vi "AndorLiveMode.vi"(8 "error in (no error)":errorcluster, 11 "Image Name":string="untitled") -> (0 "error out":errorcluster, 3 "Image":T1(plugin-control))   [LabVIEW 2018]
uses:
  <vilib>/vision/NI_Vision_Development_Module.lvlib
  <userlib>/Andor SDK/Andor SDK.lvlib
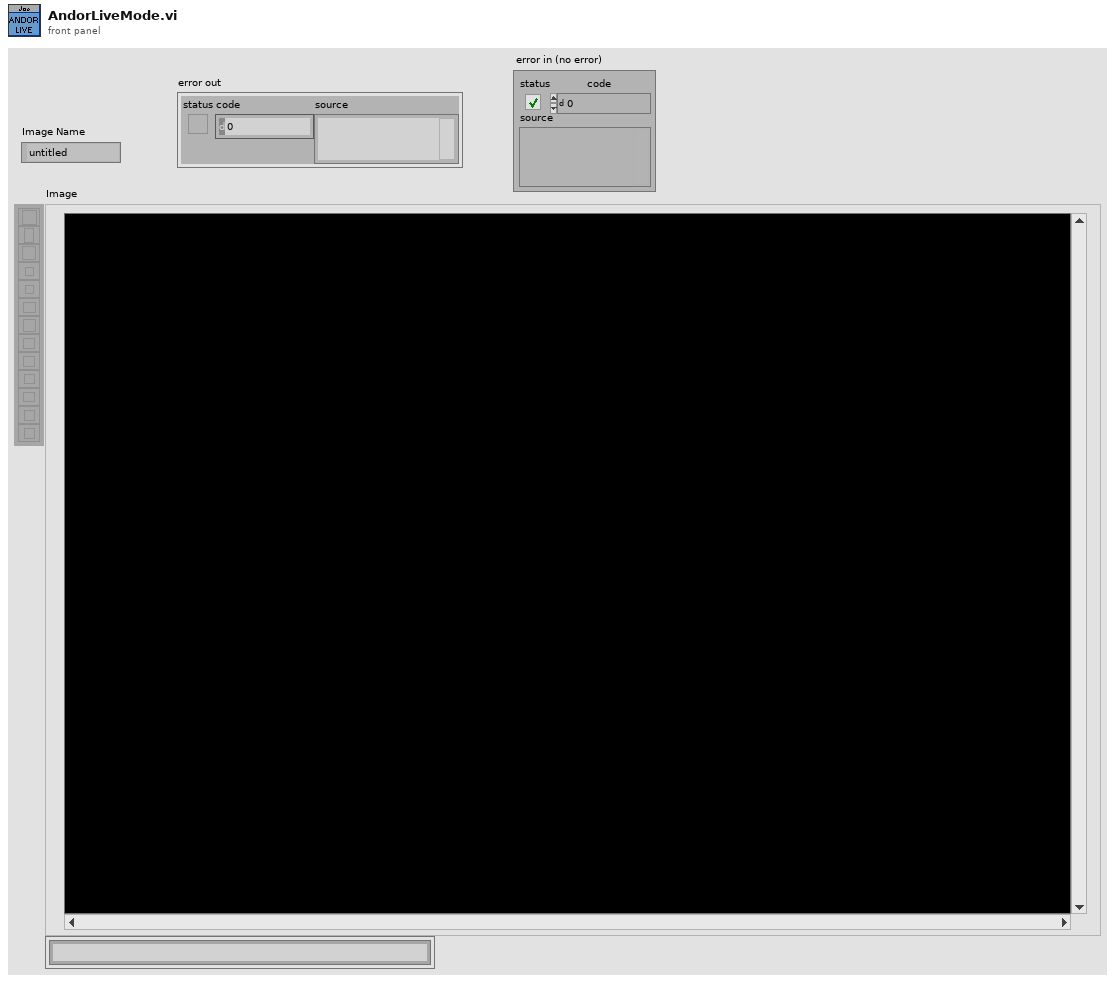
[diagram p1: front panel]
types:
  T1 = typedef "IMAQ Image.ctl" = refnum<image>
  T2 = typedef "Image Type" = u32
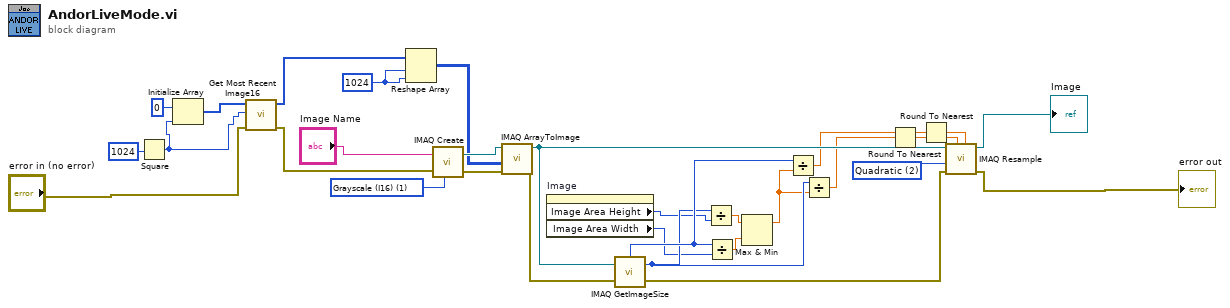
[diagram p0: block diagram]
diagram:
  w13 = u32 2 items=["Zero Order", "Bi-Linear", "Quadratic", "Cubic Spline"] ("Interpolation Type")
  w25 = T2 1 items=["Grayscale (U8)", "Grayscale (I16)", "Grayscale (SGL)", "Complex (CSG)", "RGB (U32)", "HSL (U32)", "RGB (U64)", "Grayscale (U16)"] ("Image Type")
  w26 = 1024 ("dimension size")
  n1 = Square(x=1024) -> (x^2=w11:i32)
  n2 = Initialize Array(0 ("element"), w11) -> (w8:i32[])
  n3 = call <userlib>:"Get Most Recent Image16.vi"("error in (no error)"="error in (no error)", "size"=w11, "arr"=w8) -> ("error out"=w10:errorcluster, "arr out"=w9:u16[])  [unwired: 6 in, 1 out]
  n4 = Reshape Array(w9, w26, w26) -> (w22:u16[][])
  n5 = call "IMAQ Create"("Image Name"="Image Name", "Image Type"=w25, "error in (no error)"=w10) -> ("New Image"=w24:T1, "error out"=w23:errorcluster)  [unwired: 2 in]
  n6 = call "IMAQ ArrayToImage"("error in (no error)"=w23, "Image Pixels (I16)"=w22, "Image"=w24) -> ("error out"=w19:errorcluster, "Image Out"=w15:T1)  [unwired: 7 in]
  n7 = property on="Image" class="ImageControl"() -> ("Image Area Height"=w5:u32, "Image Area Width"=w12:u32)  [unwired: 2 in, 2 out]
  n8 = call "IMAQ GetImageSize"("Image"=w15, "error in (no error)"=w19) -> ("Y Resolution"=w17:i32, "X Resolution"=w18:i32, "error out"=w14:errorcluster)  [unwired: 2 in]
  n9 = Divide(x=w17, y=w5) -> (x/y=w21:dbl)
  n10 = Divide(x=w18, y=w12) -> (x/y=w20:dbl)
  n11 = Max & Min(x=w21, y=w20) -> (max(x,y)=w16:dbl)  [unwired: 1 out]
  n12 = Divide(x=w18, y=w16) -> (x/y=w3:dbl)
  n13 = Divide(x=w17, y=w16) -> (x/y=w4:dbl)
  n14 = Round To Nearest(number=w4) -> (nearest integer value=w1:dbl)
  n15 = Round To Nearest(number=w3) -> (nearest integer value=w2:dbl)
  n16 = call "IMAQ Resample"("X Resolution"=w2, "Y Resolution"=w1, "error in (no error)"=w14, "Interpolation Type"=w13, "Image Src"=w15) -> ("error out"=→"error out":errorcluster, "Image Dst Out"=→"Image":T1)  [unwired: 5 in]
